vi "Actor Core.vi"(8 "error in":errorcluster, 11 "O3 Frequency Train Actor in":refnum<class "O3 Frequency Train Actor.lvclass">) -> (0 "error out":errorcluster, 3 "Actor out":refnum<class "Actor.lvclass">)   [LabVIEW 2014, in "Calibration.lvlib" / "O3 Frequency Train Actor.lvclass"]
doc: "(<B>Filename</B>: Actor Framework.lvlib:Actor.lvclass:Actor Core.vi)\n\nReceives messages to the actor, reacts to them, and initiates any error handling that may shut the actor down.\n\nDescendant classes may override this VI to append parallel tasks for the actor to complete while it handles messages. Overrides use the Call Parent Method node."
uses:
  O3 Frequency Train Actor.lvclass
  <vilib>/ActorFramework/Actor/Actor.lvclass
  SuperActor/Ex Nested.lvclass
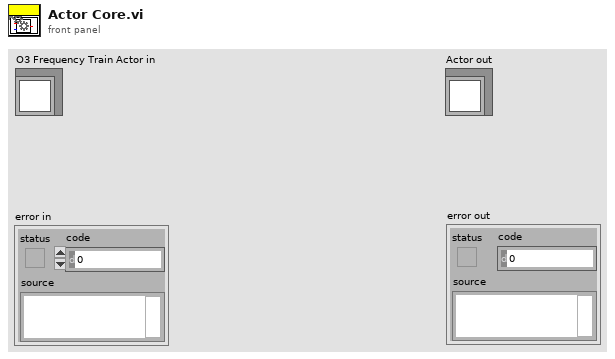
[diagram p1: front panel]
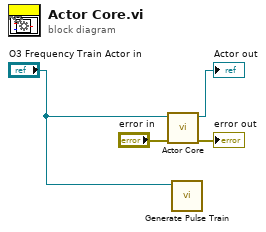
[diagram p0: block diagram]
diagram:
  n1 = call-parent "Actor Core.vi"("error in"="error in", "Actor in"="O3 Frequency Train Actor in") -> ("error out"=→"error out":errorcluster, "Actor out"=→"Actor out":refnum<class "Actor.lvclass">)  [unwired: 8 in]
  n2 = call "Generate Pulse Train.vi"("O3 Frequency Train Actor in"="O3 Frequency Train Actor in") -> ()  [unwired: 11 in]
